vi "Configure Modulation Phase Advanced.vi"(8 "error in (no error)":errorcluster, 9 "Internal Modulation Phase (0 Degree)":dbl, 10 "Channel (1: 1)":i32(ring)=1 items=["1"=1, "2"=2], 11 "VISA resource name":refnum<visa-resource-name>) -> (0 "error out":errorcluster, 3 "VISA resource name out":refnum<visa-resource-name>)   [LabVIEW 2018, in "Agilent 3352X Series.lvlib"]
doc: "Sets the phase of the internal modulation source when modulating by the internal source with shape Sine, Square, Ramp, NRamp, or Triangle.\n\n<b>Note</b>: \n(1) This VI is only applicable for 33611A, 33612A, 33621A and 33622A models and arbitrary waveforms of at least 64 samples.\n(2) This VI is intended to be used with <b>Configure Modulation (Phase).vi</b> to provide some advanced settings. Calling this VI only will not change current waveform function."
uses:
  <instrlib>/Agilent 3352X Series/Agilent 3352X Series.lvlib
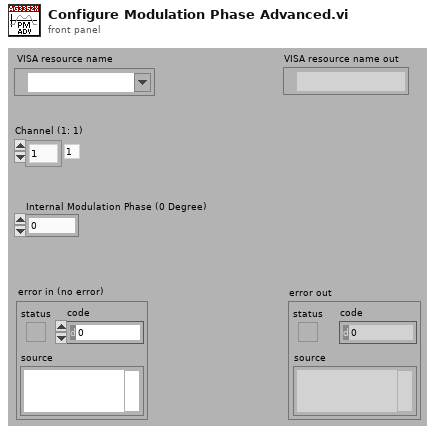
[diagram p1: front panel]
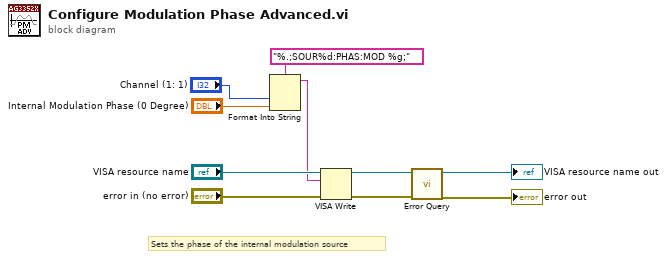
[diagram p0: block diagram]
diagram:
  # "Sets the phase of the internal modulation source"
  n1 = Format Into String(format string="%.;SOUR%d:PHAS:MOD %g;", "Channel (1: 1)", "Internal Modulation Phase (0 Degree)") -> (resulting string=w1:string)  [unwired: 2 in, 1 out]
  n2 = VISA Write(VISA resource name="VISA resource name", write buffer=w1, error in (no error)="error in (no error)") -> (VISA resource name out=w8:refnum<visa-resource-name>, error out=w7:errorcluster)  [unwired: 1 out]
  n3 = call <instrlib>:"Error Query.vi"("error in (no error)"=w7, "VISA resource name"=w8) -> ("error out"=→"error out":errorcluster, "VISA resource name out"=→"VISA resource name out":refnum<visa-resource-name>)  [unwired: 8 out]
